vi "Query Reading Buffer Data Characteristics.vi"(0 "VISA resource name":refnum<visa-resource-name>, 5 "Reading Buffer (smua.nvbuffer1)":string="smua.nvbuffer1", 7 "Data Index (1)":i32=1, 11 "error in (no error)":errorcluster) -> (3 "Measurement Range":dbl, 4 "VISA resource name out":refnum<visa-resource-name>, 6 "Measurement Function":string, 8 "Source Output State":string, 10 "Source Function":string, 14 "Source Range":dbl, 15 "error out":errorcluster)   [LabVIEW 2019, in "Keithley 2600 Series.lvlib"]
doc: "Returns the characteristics of the readings stored in a specified reading buffer."
uses:
  Keithley 2600 Series.lvlib
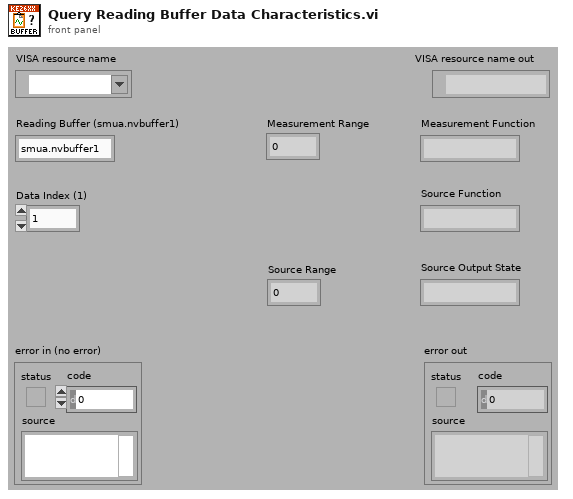
[diagram p1: front panel]
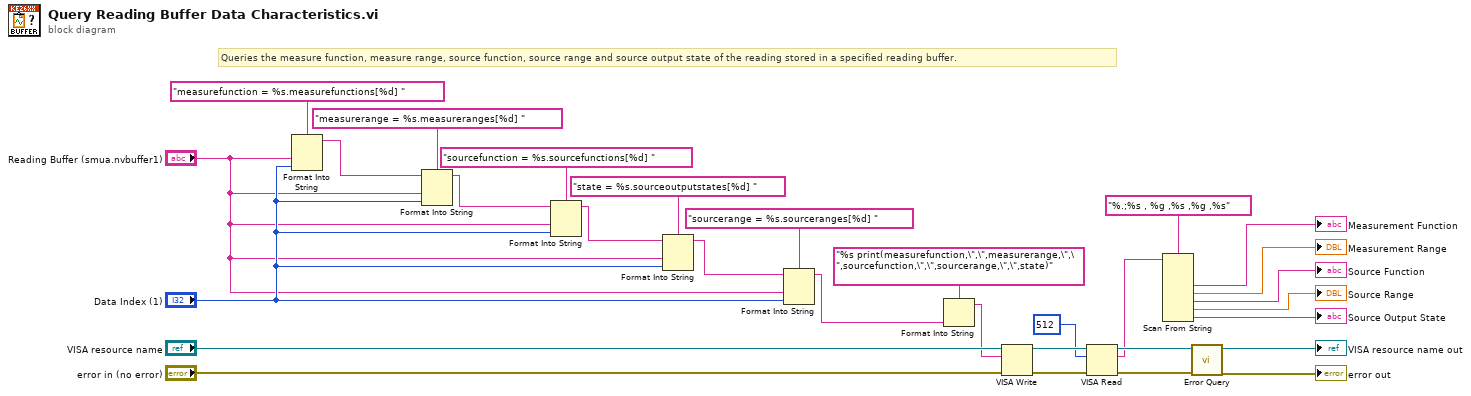
[diagram p0: block diagram]
diagram:
  # "Queries the measure function, measure range, source function, source range and source output state of the reading stored in a specified reading buffer."
  n1 = Format Into String(format string="measurefunction = %s.measurefunctions[%d] ", "Reading Buffer (smua.nvbuffer1)", "Data Index (1)") -> (resulting string=w21:string)  [unwired: 2 in, 1 out]
  n2 = Format Into String(format string="measurerange = %s.measureranges[%d] ", initial string=w21, "Reading Buffer (smua.nvbuffer1)", "Data Index (1)") -> (resulting string=w20:string)  [unwired: 1 in, 1 out]
  n3 = Format Into String(format string="sourcefunction = %s.sourcefunctions[%d] ", initial string=w20, "Reading Buffer (smua.nvbuffer1)", "Data Index (1)") -> (resulting string=w19:string)  [unwired: 1 in, 1 out]
  n4 = Format Into String(format string="state = %s.sourceoutputstates[%d] ", initial string=w19, "Reading Buffer (smua.nvbuffer1)", "Data Index (1)") -> (resulting string=w1:string)  [unwired: 1 in, 1 out]
  n5 = Format Into String(format string="sourcerange = %s.sourceranges[%d] ", initial string=w1, "Reading Buffer (smua.nvbuffer1)", "Data Index (1)") -> (resulting string=w17:string)  [unwired: 1 in, 1 out]
  n6 = Format Into String(format string="%s print(measurefunction,\",\",measurerange,\",\",sourcefunction,\",\",sourcerange,\",\",state)", w17) -> (resulting string=w15:string)  [unwired: 2 in, 1 out]
  n7 = VISA Write(VISA resource name="VISA resource name", write buffer=w15, error in (no error)="error in (no error)") -> (VISA resource name out=w14:refnum<visa-resource-name>, error out=w13:errorcluster)  [unwired: 1 out]
  n8 = VISA Read(VISA resource name=w14, byte count=u32 512, error in (no error)=w13) -> (VISA resource name out=w12:refnum<visa-resource-name>, read buffer=w9:string, error out=w11:errorcluster)  [unwired: 1 out]
  n9 = Scan From String(format string="%.;%s , %g ,%s ,%g ,%s", input string=w9) -> (output 1=→"Measurement Function":string, output 2=→"Measurement Range":dbl, output 3=→"Source Function":string, output 4=→"Source Range":dbl, output 5=→"Source Output State":string)  [unwired: 7 in, 3 out]
  n10 = call "Error Query.vi"("error in (no error)"=w11, "VISA resource name"=w12) -> ("error out"=→"error out":errorcluster, "VISA resource name out"=→"VISA resource name out":refnum<visa-resource-name>)  [unwired: 6 in, 2 out]
